vi "Plugin Main - Desaccade time data.vi"(7 "Background Mode":bool, 9 "threshold":dbl(slide) scale=0.0..500.0, 11 "Shared Data from EMA":T2={"Impulse Positions"=[], "Parameter Impuls Series"=[], "Data File"={"Data Channels"=[], "Sample Rate"=0, "Channel List"=[]}, "desacc "={"Threshold 1 [Acc]"=7000.0, "Threshold 2 [% of TH1]"=60, "tolerance"=3, "Search WD "=0.1, " always use TH2"=FALSE, "Range"=2.0, "Max time"=120.0, "Min time"=20.0, "Velocity Threshold"=150}, "Experiment Parameters 2"={"Subject"="", "Strain"="", "Rotation plane"="", "Experimenter"="", "Trial"=0.0, "Time"=0.0}} {"Parameter Impuls Series"."Gain" format="%.1f"; "Parameter Impuls Series"."Offset" format="%.1f"}) -> (3 "Shared Data from EMA 2":T2={"Impulse Positions"=[], "Parameter Impuls Series"=[], "Data File"={"Data Channels"=[], "Sample Rate"=0, "Channel List"=[]}, "desacc "={"Threshold 1 [Acc]"=7000.0, "Threshold 2 [% of TH1]"=60, "tolerance"=3, "Search WD "=0.1, " always use TH2"=FALSE, "Range"=2.0, "Max time"=120.0, "Min time"=20.0, "Velocity Threshold"=150}, "Experiment Parameters 2"={"Subject"="", "Strain"="", "Rotation plane"="", "Experimenter"="", "Trial"=0.0, "Time"=0.0}} {"Parameter Impuls Series"."Gain" format="%.1f"; "Parameter Impuls Series"."Offset" format="%.1f"})   [LabVIEW 2016]
uses:
  Plugin Shared Data.ctl
  core/type-defs/TD_Impulse Parameter.ctl
  <vilib>/Analysis/1siggen.llb/Ramp Pattern by Samples.vi
  <vilib>/Analysis/NI_AALBase.lvlib
  <vilib>/ptbypt/NI_PtbyPt.lvlib
  core/core.lvlib
  plugin data.lvlib
panel:
  out "XY Graph":T1(graph)
  in  "min delta Position for Quick-Phase":dbl=0.01
  in  "+/- # points post":i32
  in  "Time [ms]":dbl=60.0
  in  "Preview delete":bool
  in  "+/- # points pre":i32
  in  "Eye":enum16{"Right", "Left"}(ring)=enum."Left"
  in  "Pos/Vel":enum16{"Position", "Velocity"}(ring)=enum."Velocity"
  in  "Stop Button":bool
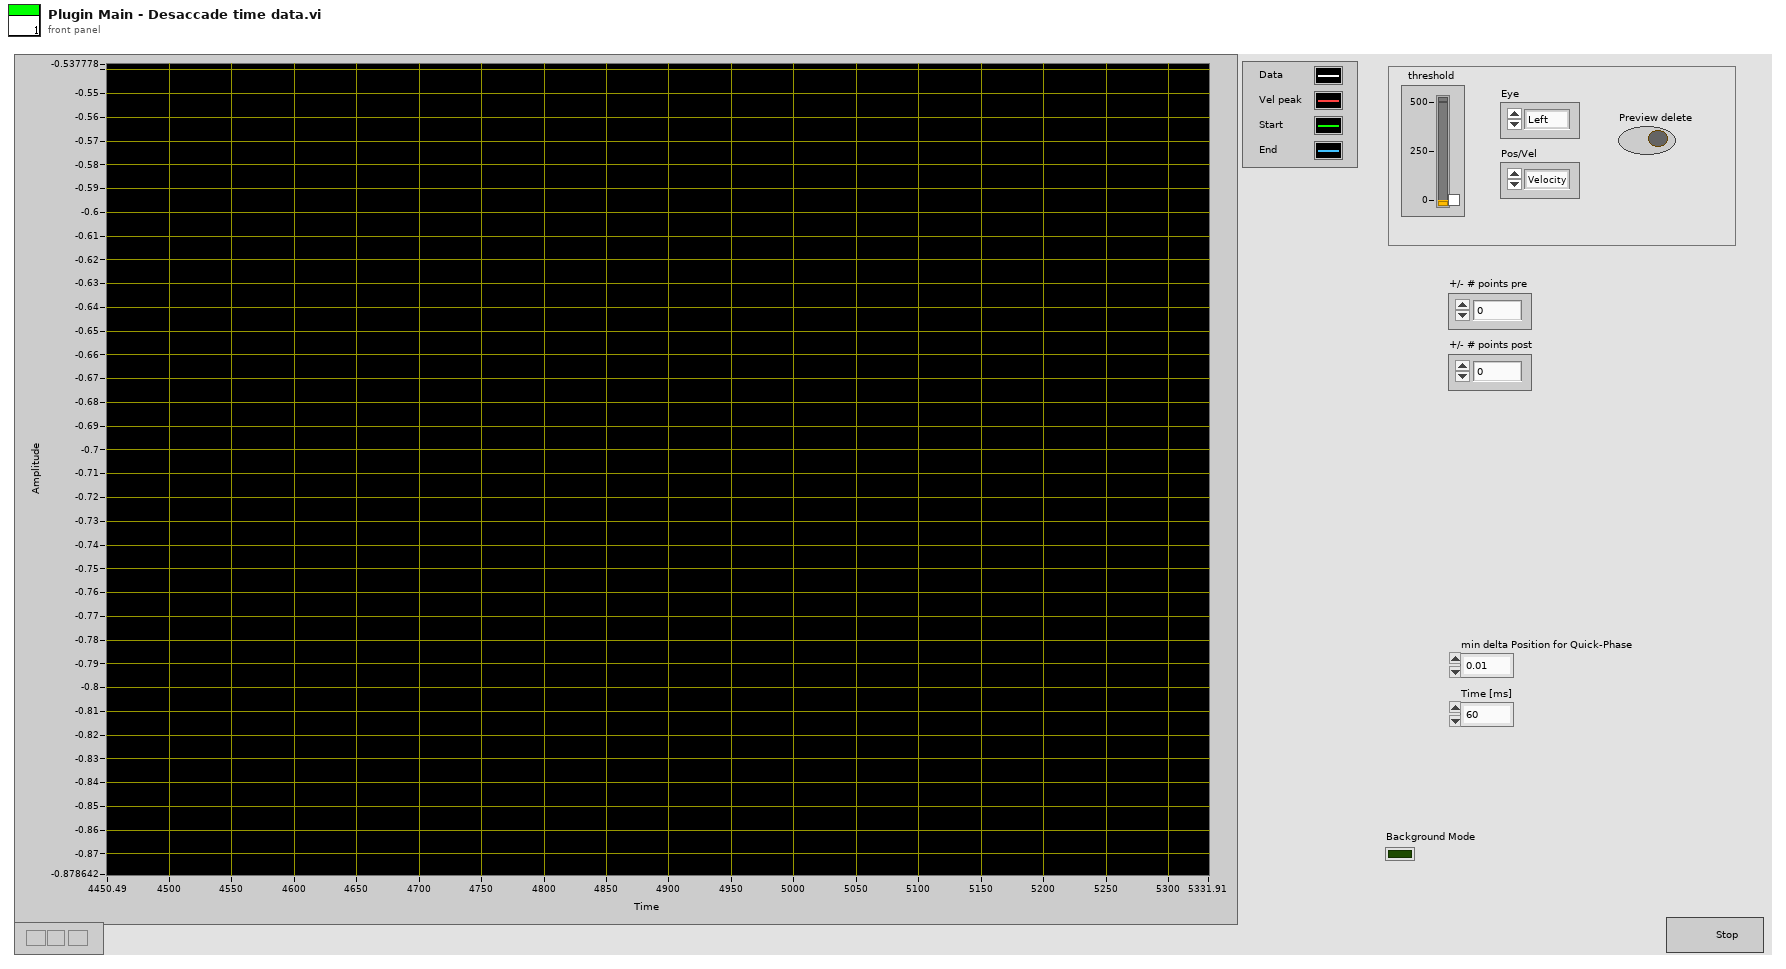
[diagram p1: front panel]
types:
  T1 = cluster{"Ramp Pattern":dbl[], "Data Channels":dbl[]}[]
  T2 = typedef "plugin data.lvlib/Plugin Shared Data.ctl" = cluster{"Impulse Positions":cluster{"Start":i32, "End":i32, "Impulse Plane":enum16{"Other", "Yaw", "Pitch", "Roll", "LARP", "RALP"}, "Impulse Direction +ve?":bool, "Time offset":i32, "Amplitude offset":dbl}[], "Parameter Impuls Series":T3, "Data File":cluster{"Data Channels":dbl[][], "Sample Rate":i32, "Channel List":string[]}, "desacc ":cluster{"Threshold 1 [Acc]":dbl, "Threshold 2 [% of TH1]":i32, "tolerance":i32, "Search WD ":dbl, " always use TH2":bool, "Range":dbl, "Max time":dbl, "Min time":dbl, "Velocity Threshold":i32}, "Experiment Parameters 2":cluster{"Subject":string, "Strain":string, "Rotation plane":string, "Experimenter":string, "Trial":dbl, "Time":dbl}}
  T3 = typedef "core.lvlib/TD_Impulse Parameter.ctl" = cluster{"Color":u32, "Visible":bool, "Channel":u16, "Invert":bool, "Desaccade":bool, "Offset":dbl, "Gain":dbl}[]
  T4 = cluster{"Channel Groups":i32[][][], "Saccade pos tmp":i32[], "Saccade dir":bool[], "newData":dbl[][], "Eye":enum16{"Right", "Left"}, "Saccade start tmp":i32[], "Saccade end tmp":i32[], "Saccades R":cluster{"Saccade pos":i32[], "Saccade start":i32[], "Saccade end":i32[]}, "Saccades L":cluster{"Saccade pos":i32[], "Saccade start":i32[], "Saccade end":i32[]}}
  T5 = cluster{"Ramp Pattern":dbl[], "Data Channels":dbl[]}
  T6 = cluster{"+/- # points pre":i32, "+/- # points post":i32, "threshold":dbl}
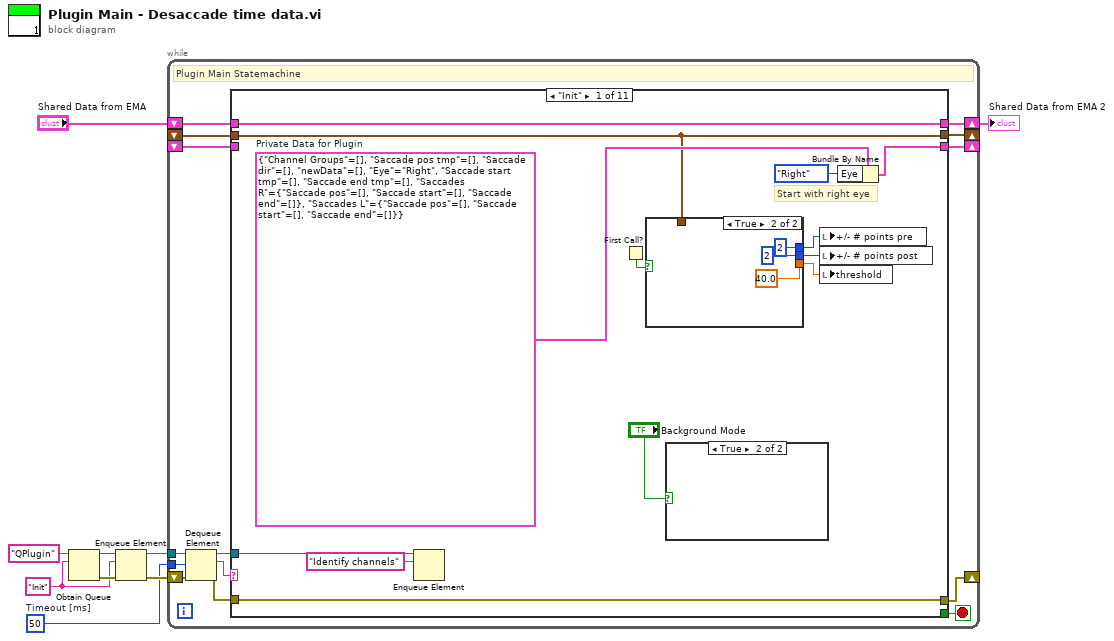
[diagram p0: block diagram]
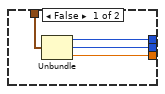
[diagram p2: hidden frame]
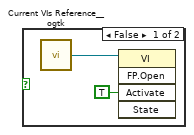
[diagram p3: hidden frame]
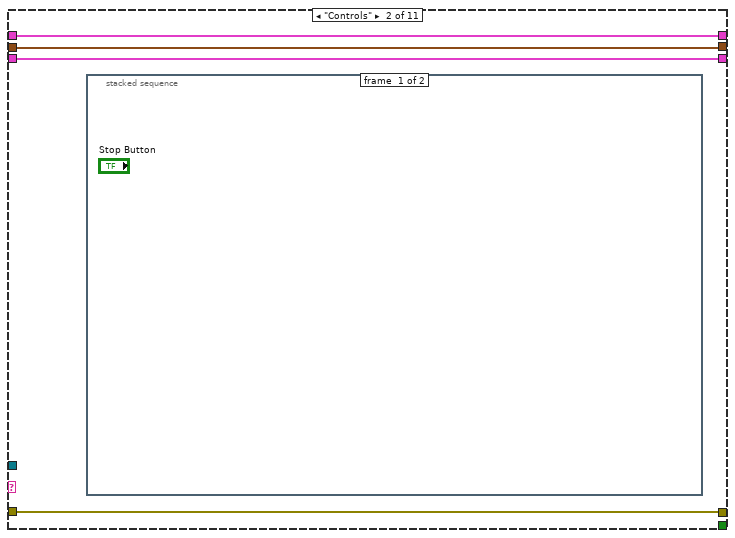
[diagram p4: hidden frame]
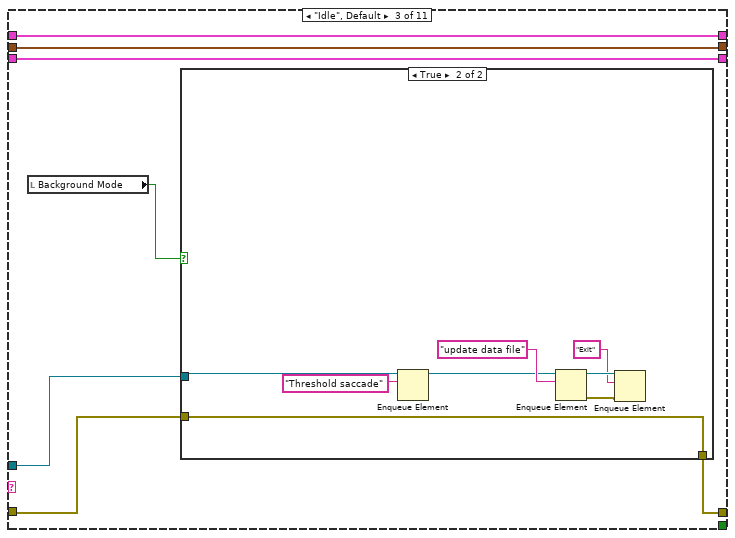
[diagram p6: hidden frame]
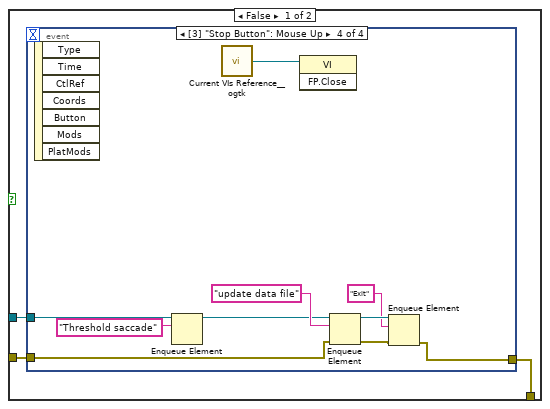
[diagram p7: hidden frame]
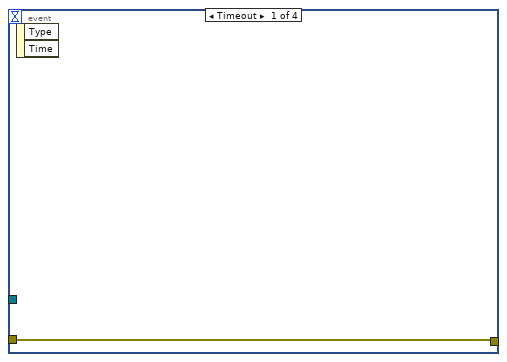
[diagram p8: hidden frame]
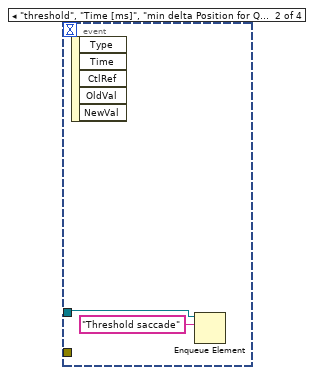
[diagram p9: hidden frame]
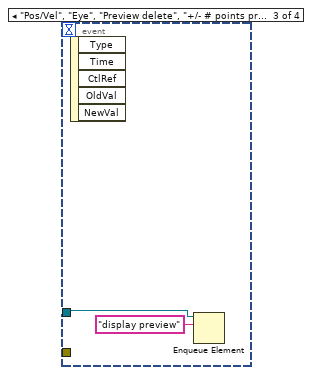
[diagram p10: hidden frame]
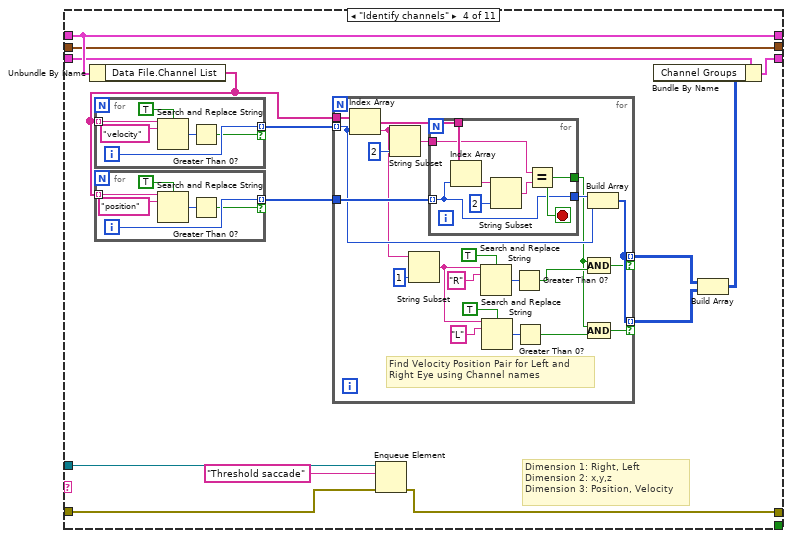
[diagram p11: hidden frame]
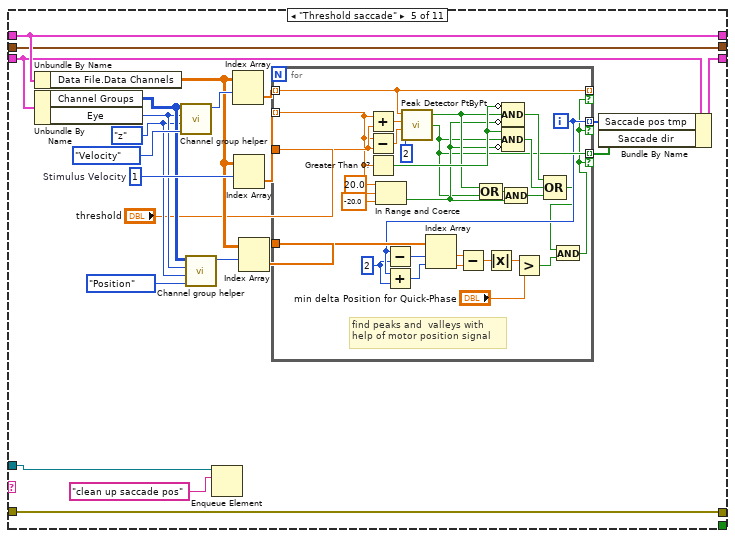
[diagram p12: hidden frame]
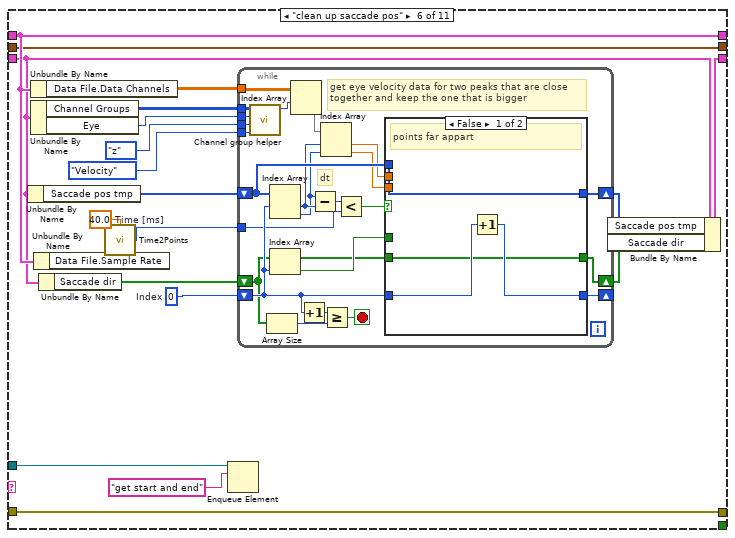
[diagram p13: hidden frame]
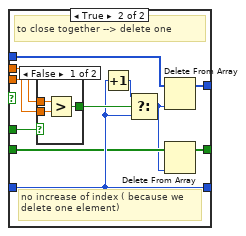
[diagram p14: hidden frame]
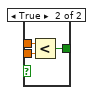
[diagram p15: hidden frame]
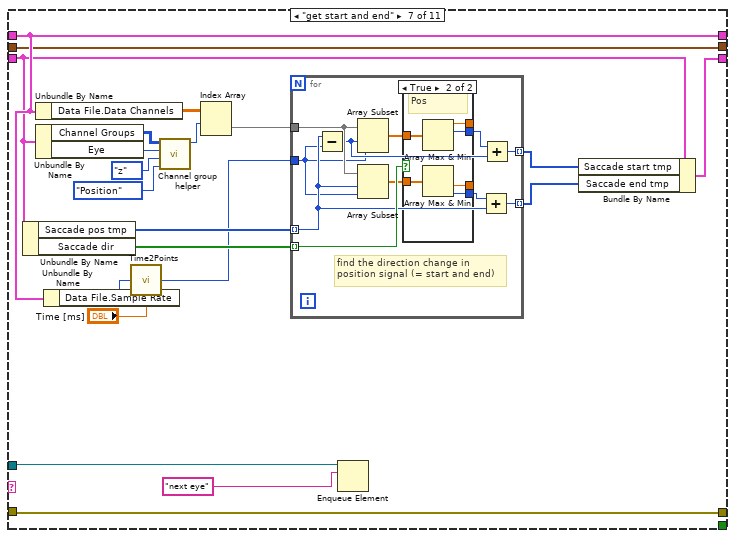
[diagram p16: hidden frame]
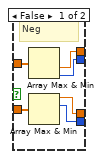
[diagram p17: hidden frame]
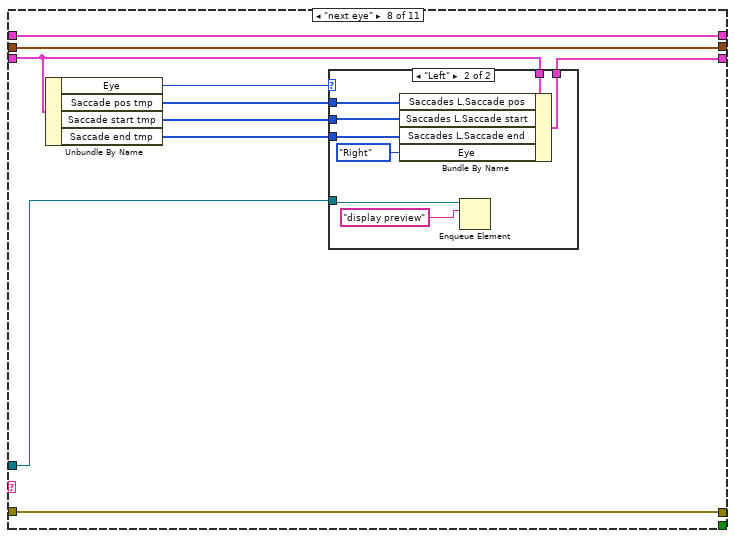
[diagram p18: hidden frame]
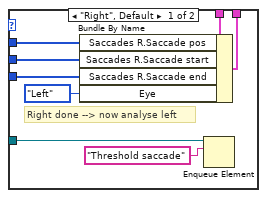
[diagram p19: hidden frame]
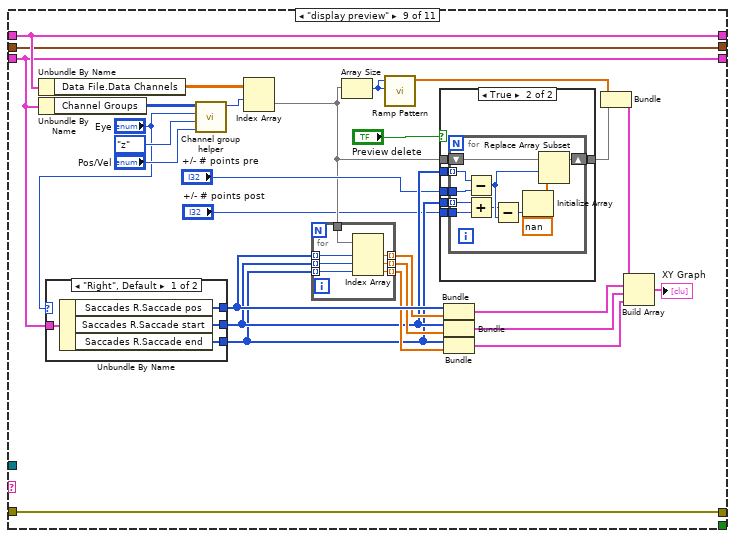
[diagram p20: hidden frame]
diagram:
  w3 = 50  # Timeout [ms]
  w7 = "Init"
  n1 = Obtain Queue(name (unnamed)="QPlugin", element data type=w7) -> (queue out=w8:refnum<queue>, error out=w9:errorcluster)  [unwired: 3 in, 1 out]
  n2 = Enqueue Element(queue=w8, element=w7, error in (no error)=w9) -> (queue out=w5:refnum<queue>, error out=w4:errorcluster)  [unwired: 1 in, 1 out]
  n3 = while {
    tunnel: w5 -> [w22]
    tunnel: w3 -> [w20]
    shift-right: [w16] -> _
    shift-left: w4 -> [w21]
    shift-right: [w15] -> _
    shift-left: _ -> [w14]
    shift-right: [w12] -> w1
    shift-left: "Shared Data from EMA" -> [w13]
    shift-right: [w11] -> _
    shift-left: _ -> [w10]
    stop <- w23 stop-if-true
    # "Plugin Main Statemachine"
    n4 = Dequeue Element(queue=w22, timeout in ms (-1)=w20, error in (no error)=w21) -> (queue out=w19:refnum<queue>, element=w18:string, error out=w17:errorcluster)  [unwired: 1 out]
    n5 = case shown="\"Init\"" w18 {
      tunnel: [_ _ _ _ _ _ _ _ _ _ w451] -> w23
      tunnel: w19 -> [w35 _ w54 w86 w154 w205 w256 w298 _ _ _]
      tunnel: w17 -> [w36 w47 w53 w85 w158 w207 w273 w305 w350 w391 w450]
      tunnel: [w36 w47 w52 w84 w158 w207 w273 w305 w350 w391 w450] -> w16
      tunnel: [w32 w48 w56 w88 w155 w199 w258 w299 w343 w388 w449] -> w15
      tunnel: w14 -> [_ w48 w56 w89 w156 w191 w259 w300 w343 w388 w449]
      tunnel: w13 -> [w30 w49 w55 w96 w157 w195 w263 w306 w349 w387 w448]
      tunnel: [w30 w49 w55 w96 w157 w195 w263 w306 w349 w386 w448] -> w12
      tunnel: [w25 w46 w50 w83 w137 w188 w253 w297 w323 w384 w444] -> w11
      tunnel: w10 -> [w25 w46 w50 w83 w137 w188 w253 w297 w323 w384 _]
      frame "Init" {
        w33 = T4 {"Channel Groups"=[], "Saccade pos tmp"=[], "Saccade dir"=[], "newData"=[], "Eye"=enum."Right", "Saccade start tmp"=[], "Saccade end tmp"=[], "Saccades R"={"Saccade pos"=[], "Saccade start"=[], "Saccade end"=[]}, "Saccades L"={"Saccade pos"=[], "Saccade start"=[], "Saccade end"=[]}}  # Private Data for Plugin
        # "Start with right eye"
        n6 = Enqueue Element(queue=w35, element="Identify channels") -> ()  [unwired: 2 in, 3 out]
        n7 = First Call?() -> (First Call?: T/F=w24:bool)
        n8 = case shown="True" w24 {
          tunnel: [w40 2 ("+/- # points pre")] -> w28
          tunnel: [w39 2 ("+/- # points post")] -> w27
          tunnel: [w38 40.0 ("threshold")] -> w26
          tunnel: w25 -> [w37 _]
          frame False {
            n9 = Unbundle(w37) -> ("+/- # points pre"=w40:i32, "+/- # points post"=w39:i32, "threshold"=w38:dbl)
          }
          frame True {
          }
        }
        n10 = case shown="True" "Background Mode" {
          frame False {
            n11 = call <userlib>:"Current VIs Reference__ogtk.vi"() -> ("Current VI's reference"=w45:refnum<vi>)  [unwired: 5 in]
            n12 = invoke class="VI" method="FP.Open"(reference=w45, "Activate"=TRUE ("Activate?")) -> ()  [unwired: 3 in, 5 out]
          }
          frame True {
          }
        }
        n13 = local write "+/- # points pre"(w28) -> ()
        n14 = local write "+/- # points post"(w27) -> ()
        n15 = local write "threshold"(w26) -> ()
        n16 = Bundle By Name(cluster=w33, "Eye"=enum16{"Right", "Left"}."Right") -> (w32:T4)
      }
      frame "Controls" {
        n17 = stacked-sequence {
          frame #0 {
          }
          frame #1 {
          }
        }
      }
      frame "Idle", Default {
        n18 = local read "Background Mode"() -> (w51:bool)
        n19 = case shown="True" w51 {
          tunnel: w54 -> [w59 w75]
          tunnel: w53 -> [w58 w82]
          tunnel: [w57 w82] -> w52
          frame False {
            n20 = event shown="[3] \"Stop Button\": Mouse Up" {
              selector: _ -> [_ _ _ _]
              dyn-events: _ -> [_ _ _ _]
              timeout: _ -> [_ _ _ _]
              tunnel: w59 -> [_ w61 w63 w67]
              tunnel: w58 -> [w60 _ _ w73]
              tunnel: [w60 _ _ w70] -> w57
              event Timeout {
                n21 = event-data() -> ()  [unwired: 1 in, 2 out]
              }
              event "threshold", "Time [ms]", "min delta Position for Quick-Phase": Value Change {
                n22 = event-data() -> ()  [unwired: 1 in, 5 out]
                n23 = Enqueue Element(queue=w61, element="Threshold saccade") -> ()  [unwired: 2 in, 3 out]
              }
              event "Pos/Vel", "Eye", "Preview delete", "+/- # points pre", "+/- # points post": Value Change {
                n24 = event-data() -> ()  [unwired: 1 in, 5 out]
                n25 = Enqueue Element(queue=w63, element="display preview") -> ()  [unwired: 2 in, 3 out]
              }
              event "Stop Button": Mouse Up {
                n26 = event-data() -> ()  [unwired: 1 in, 7 out]
                n27 = Enqueue Element(queue=w67, element="Threshold saccade") -> (queue out=w66:refnum<queue>)  [unwired: 2 in, 2 out]
                n28 = call <userlib>:"Current VIs Reference__ogtk.vi"() -> ("Current VI's reference"=w65:refnum<vi>)  [unwired: 5 in]
                n29 = invoke class="VI" method="FP.Close"(reference=w65) -> ()  [unwired: 2 in, 3 out]
                n30 = Enqueue Element(queue=w66, element="update data file", error in (no error)=w73) -> (queue out=w72:refnum<queue>, error out=w71:errorcluster)  [unwired: 1 in, 1 out]
                n31 = Enqueue Element(queue=w72, element="Exit", error in (no error)=w71) -> (error out=w70:errorcluster)  [unwired: 1 in, 2 out]
              }
            }
          }
          frame True {
            n32 = Enqueue Element(queue=w75, element="Threshold saccade") -> (queue out=w76:refnum<queue>)  [unwired: 2 in, 2 out]
            n33 = Enqueue Element(queue=w76, element="update data file") -> (queue out=w80:refnum<queue>, error out=w79:errorcluster)  [unwired: 2 in, 1 out]
            n34 = Enqueue Element(queue=w80, element="Exit", error in (no error)=w79) -> ()  [unwired: 1 in, 3 out]
          }
        }
      }
      frame "Identify channels" {
        # "Dimension 1: Right, Left\nDimension 2: x,y,z\nDimension 3: Position, Velocity"
        n35 = Unbundle By Name(w96) -> ("Data File.Channel List"=w93:string[])
        n36 = for {
          tunnel: w93 -> [w136] mode=indexing
          tunnel: [w133] -> w95 mode=indexing if=w132
          i -> [w133]
          n37 = Search and Replace String(case sensitive?=TRUE ("ignore case? (F)"), input string=w136, search string="velocity") -> (number of replacements=w134:i32)  [unwired: 5 in, 3 out]
          n38 = Greater Than 0?(x=w134) -> (x > 0?=w132:bool)
        }
        n39 = for {
          tunnel: w93 -> [w130] mode=indexing
          tunnel: [w127] -> w94 mode=indexing if=w126
          i -> [w127]
          n40 = Search and Replace String(case sensitive?=TRUE ("ignore case? (F)"), input string=w130, search string="position") -> (number of replacements=w128:i32)  [unwired: 5 in, 3 out]
          n41 = Greater Than 0?(x=w128) -> (x > 0?=w126:bool)
        }
        n42 = for {
          tunnel: w95 -> [w112] mode=indexing
          tunnel: w93 -> [w116]
          tunnel: w94 -> [w117]
          tunnel: [w108] -> w92 mode=indexing if=w98
          tunnel: [w108] -> w91 mode=indexing if=w97
          # "Find Velocity Position Pair for Left and \nRight Eye using Channel names"
          n43 = Index Array(array=w116, index=w112) -> (element=w100:string)
          n44 = String Subset(string=w100, length (rest)=2 ("length (rest)")) -> (substring=w114:string)  [unwired: 1 in]
          n45 = String Subset(string=w100, length (rest)=1 ("length (rest)")) -> (substring=w104:string)  [unwired: 1 in]
          n46 = for {
            tunnel: w117 -> [w118] mode=indexing
            tunnel: w116 -> [w123]
            tunnel: w114 -> [w120]
            tunnel: [w119] -> w102
            tunnel: [w118] -> w113
            stop <- w119 stop-if-true
            n47 = Index Array(array=w123, index=w118) -> (element=w124:string)
            n48 = String Subset(string=w124, length (rest)=2 ("length (rest)")) -> (substring=w121:string)  [unwired: 1 in]
            n49 = Equal?(x=w120, y=w121) -> (x = y?=w119:bool)
          }
          n50 = Search and Replace String(case sensitive?=TRUE ("ignore case? (F)"), input string=w104, search string="R") -> (number of replacements=w109:i32)  [unwired: 5 in, 3 out]
          n51 = Search and Replace String(case sensitive?=TRUE ("ignore case? (F)"), input string=w104, search string="L") -> (number of replacements=w107:i32)  [unwired: 5 in, 3 out]
          n52 = Greater Than 0?(x=w109) -> (x > 0?=w103:bool)
          n53 = Greater Than 0?(x=w107) -> (x > 0?=w101:bool)
          n54 = Build Array(w113, w112) -> (w108:i32[])
          n55 = Compound Arithmetic op=AND(w102, w103) -> (w98:bool)
          n56 = Compound Arithmetic op=AND(w102, w101) -> (w97:bool)
        }
        n57 = Enqueue Element(queue=w86, element="Threshold saccade", error in (no error)=w85) -> (error out=w84:errorcluster)  [unwired: 1 in, 2 out]
        n58 = Build Array(w92, w91) -> (w90:i32[][][])
        n59 = Bundle By Name(cluster=w89, "Channel Groups"=w90) -> (w88:T4)
      }
      frame "Threshold saccade" {
        w140 = enum16{"x", "y", "z"}."z" ("Eye component")
        w151 = 1  # Stimulus Velocity
        n60 = Unbundle By Name(w157) -> ("Data File.Data Channels"=w145:dbl[][])
        n61 = Unbundle By Name(w156) -> ("Channel Groups"=w142:i32[][][], "Eye"=w141:enum16{"Right", "Left"})
        n62 = call "Channel group helper.vi"("Pos/Vel"=enum16{"Position", "Velocity"}."Velocity", "Eye component"=w140, "Eye"=w141, "Channel Groups"=w142) -> ("Channel"=w149:i32)  [unwired: 7 in]
        n63 = call "Channel group helper.vi"("Pos/Vel"=enum16{"Position", "Velocity"}."Position", "Eye component"=w140, "Eye"=w141, "Channel Groups"=w142) -> ("Channel"=w144:i32)  [unwired: 7 in]
        n64 = Enqueue Element(queue=w154, element="clean up saccade pos") -> ()  [unwired: 2 in, 3 out]
        n65 = Index Array(array=w145, index (row)=w149) -> (element=w147:dbl[])  [unwired: 1 in]
        n66 = Index Array(array=w145, index (row)=w151) -> (element=w146:dbl[])  [unwired: 1 in]
        n67 = Index Array(array=w145, index (row)=w144) -> (element=w143:dbl[])  [unwired: 1 in]
        n68 = for {
          tunnel: w147 -> [w187] mode=indexing
          tunnel: w146 -> [w180] mode=indexing
          tunnel: "threshold" -> [w184]
          tunnel: [w187] -> _ mode=indexing if=w159
          tunnel: [w170] -> w150 mode=indexing if=w159
          tunnel: [w172] -> w152 mode=indexing if=w159
          tunnel: w143 -> [w171]
          i -> [w170]
          w169 = 2 ("y")
          # "find peaks and  valleys with \nhelp of motor position signal"
          n69 = Add(x=w180, y=w184) -> (x+y=w183:dbl)
          n70 = Subtract(x=w180, y=w184) -> (x-y=w182:dbl)
          n71 = Greater Than 0?(x=w180) -> (x > 0?=w177:bool)
          n72 = In Range and Coerce(upper limit=20.0, x=w180, lower limit=-20.0) -> (In Range?=w174:bool)  [unwired: 1 out]
          n73 = Subtract(x=w170, y=w169) -> (x-y=w168:i32)
          n74 = Add(x=w170, y=w169) -> (x+y=w167:i32)
          n75 = call <vilib>:"Peak Detector PtByPt.vi"("x"=w187, "threshold peak"=w183, "threshold valley"=w182, "width"=2) -> ("peak"=w176:bool, "valley"=w172:bool)  [unwired: 1 in, 1 out]
          n76 = Index Array(array=w171, index #1=w168, index #2=w167) -> (element #1=w166:dbl, element #2=w165:dbl)
          n77 = Subtract(x=w166, y=w165) -> (x-y=w164:dbl)
          n78 = Compound Arithmetic op=OR(w176, w172) -> (w175:bool)
          n79 = Absolute Value(x=w164) -> (abs(x)=w163:dbl)
          n80 = Compound Arithmetic op=AND(invert w177, w176, invert w174) -> (w185:bool)
          n81 = Compound Arithmetic op=AND(w177, w172, invert w174) -> (w181:bool)
          n82 = Compound Arithmetic op=AND(w175, w174) -> (w173:bool)
          n83 = Greater?(x=w163, y="min delta Position for Quick-Phase") -> (0:w160:bool)
          n84 = Compound Arithmetic op=OR(w185, w181, w173) -> (w161:bool)
          n85 = And(x=w161, y=w160) -> (x .and. y?=w159:bool)
        }
        n86 = Bundle By Name(cluster=w156, "Saccade pos tmp"=w150, "Saccade dir"=w152) -> (w155:T4)
      }
      frame "clean up saccade pos" {
        w193 = 40.0  # Time [ms]
        w203 = 0  # Index
        n87 = Unbundle By Name(w191) -> ("Saccade pos tmp"=w204:i32[])
        n88 = Unbundle By Name(w195) -> ("Data File.Data Channels"=w202:dbl[][])
        n89 = Unbundle By Name(w191) -> ("Channel Groups"=w198:i32[][][], "Eye"=w197:enum16{"Right", "Left"})
        n90 = Unbundle By Name(w195) -> ("Data File.Sample Rate"=w194:i32)
        n91 = Unbundle By Name(w191) -> ("Saccade dir"=w190:bool[])
        n92 = call "Time2Points.vi"("Time [ms]"=w193, "Sample Rate"=w194) -> ("Points"=w192:i32)  [unwired: 2 in]
        n93 = Enqueue Element(queue=w205, element="get start and end") -> ()  [unwired: 2 in, 3 out]
        n94 = while {
          shift-right: [w225] -> w201
          shift-left: w204 -> [w228]
          shift-right: [w229] -> _
          shift-left: w203 -> [w221]
          tunnel: w202 -> [w214]
          shift-right: [w223] -> w200
          shift-left: w190 -> [w219]
          tunnel: w198 -> [w213]
          tunnel: w197 -> [w210]
          tunnel: enum16{"Position", "Velocity"}."Velocity" ("Pos/Vel") -> [w212]
          tunnel: w192 -> [w220]
          tunnel: enum16{"x", "y", "z"}."z" ("Eye component") -> [w211]
          stop <- w226 stop-if-true
          # "dt"
          # "get eye velocity data for two peaks that are close\ntogether and keep the one that is bigger"
          n95 = call "Channel group helper.vi"("Pos/Vel"=w212, "Eye component"=w211, "Eye"=w210, "Channel Groups"=w213) -> ("Channel"=w209:i32)  [unwired: 7 in]
          n96 = Array Size(array=w219) -> (size(s)=w227:i32)
          n97 = Index Array(array=w228, index #1=w221) -> (element #1=w218:i32, element #2=w217:i32)  [unwired: 1 in]
          n98 = Index Array(array=w219, index=w221) -> (element=w222:bool)
          n99 = Index Array(array=w214, index (row)=w209) -> (element=w208:dbl[])  [unwired: 1 in]
          n100 = Increment(x=w221) -> (x+1=w224:i32)
          n101 = Subtract(x=w217, y=w218) -> (x-y=w231:i32)
          n102 = Index Array(array=w208, index #1=w218, index #2=w217) -> (element #1=w216:dbl, element #2=w215:dbl)
          n103 = Greater Or Equal?(x=w224, y=w227) -> (x >= y?=w226:bool)
          n104 = Less?(x=w231, y=w220) -> (x < y?=w230:bool)
          n105 = case shown="False" w230 {
            tunnel: w216 -> [_ w246]
            tunnel: w215 -> [_ w245]
            tunnel: w221 -> [w234 w240]
            tunnel: [w235 w243] -> w225
            tunnel: w228 -> [w235 w242]
            tunnel: [w233 w240] -> w229
            tunnel: w219 -> [w232 w239]
            tunnel: [w232 w238] -> w223
            tunnel: w222 -> [_ w237]
            frame False {
              # "points far appart"
              n106 = Increment(x=w234) -> (x+1=w233:i32)
            }
            frame True {
              # "no increase of index ( because we \ndelete one element)"
              # "to close together --> delete one"
              n107 = case shown="False" w237 {
                tunnel: w246 -> [w249 w252]
                tunnel: w245 -> [w248 w251]
                tunnel: [w247 w250] -> w244
                frame False {
                  n108 = Greater?(x=w249, y=w248) -> (0:w247:bool)
                }
                frame True {
                  n109 = Less?(x=w252, y=w251) -> (x < y?=w250:bool)
                }
              }
              n110 = Increment(x=w240) -> (x+1=w241:i32)
              n111 = Select(t=w241, s=w244, f=w240) -> (s? t:f=w236:i32)
              n112 = Delete From Array(array=w242, index=w236) -> (array with subset deleted=w243:i32[])  [unwired: 1 in, 1 out]
              n113 = Delete From Array(array=w239, index=w236) -> (array with subset deleted=w238:bool[])  [unwired: 1 in, 1 out]
            }
          }
        }
        n114 = Bundle By Name(cluster=w191, "Saccade pos tmp"=w201, "Saccade dir"=w200) -> (w199:T4)
      }
      frame "get start and end" {
        n115 = Unbundle By Name(w259) -> ("Saccade pos tmp"=w272:i32[], "Saccade dir"=w271:bool[])
        n116 = Unbundle By Name(w263) -> ("Data File.Data Channels"=w269:dbl[][])
        n117 = Unbundle By Name(w259) -> ("Channel Groups"=w268:i32[][][], "Eye"=w267:enum16{"Right", "Left"})
        n118 = Unbundle By Name(w263) -> ("Data File.Sample Rate"=w262:i32)
        n119 = call "Time2Points.vi"("Time [ms]"="Time [ms]", "Sample Rate"=w262) -> ("Points"=w260:i32)  [unwired: 2 in]
        n120 = call "Channel group helper.vi"("Pos/Vel"=enum16{"Position", "Velocity"}."Position", "Eye component"=enum16{"x", "y", "z"}."z", "Eye"=w267, "Channel Groups"=w268) -> ("Channel"=w265:i32)  [unwired: 7 in]
        n121 = Index Array(array=w269, index (row)=w265) -> (element=w270:dbl[])  [unwired: 1 in]
        n122 = for {
          tunnel: w272 -> [w275] mode=indexing
          tunnel: w270 -> [w279]
          tunnel: [w282] -> w255 mode=indexing
          tunnel: [w281] -> w254 mode=indexing
          tunnel: w271 -> [w278] mode=indexing
          tunnel: w260 -> [w274]
          # "find the direction change in \nposition signal (= start and end)"
          n123 = Subtract(x=w275, y=w274) -> (x-y=w276:i32)
          n124 = Array Subset(array=w279, index=w276, length=w274) -> (w284:dbl[])
          n125 = Array Subset(array=w279, index=w275, length=w274) -> (w277:dbl[])
          n126 = case shown="True" w278 {
            tunnel: w284 -> [w290 w296]
            tunnel: [w288 w291] -> w283
            tunnel: [w289 w292] -> _
            tunnel: [w286 w294] -> _
            tunnel: [w285 w293] -> w280
            tunnel: w277 -> [w287 w295]
            frame False {
              # "Neg"
              n127 = Array Max & Min(array=w290) -> (min value=w289:dbl, min index (indices)=w288:i32)  [unwired: 2 out]
              n128 = Array Max & Min(array=w287) -> (max value=w286:dbl, max index (indices)=w285:i32)  [unwired: 2 out]
            }
            frame True {
              # "Pos"
              n129 = Array Max & Min(array=w296) -> (max value=w292:dbl, max index (indices)=w291:i32)  [unwired: 2 out]
              n130 = Array Max & Min(array=w295) -> (min value=w294:dbl, min index (indices)=w293:i32)  [unwired: 2 out]
            }
          }
          n131 = Add(x=w280, y=w275) -> (x+y=w281:i32)
          n132 = Add(x=w283, y=w276) -> (x+y=w282:i32)
        }
        n133 = Enqueue Element(queue=w256, element="next eye") -> ()  [unwired: 2 in, 3 out]
        n134 = Bundle By Name(cluster=w259, "Saccade start tmp"=w255, "Saccade end tmp"=w254) -> (w258:T4)
      }
      frame "next eye" {
        n135 = Unbundle By Name(w300) -> ("Eye"=w304:enum16{"Right", "Left"}, "Saccade pos tmp"=w303:i32[], "Saccade start tmp"=w302:i32[], "Saccade end tmp"=w301:i32[])
        n136 = case shown="\"Left\"" w304 {
          tunnel: w300 -> [w314 w322]
          tunnel: w303 -> [w313 w320]
          tunnel: w302 -> [w312 w319]
          tunnel: w301 -> [w311 w318]
          tunnel: [w310 w321] -> w299
          tunnel: w298 -> [w308 w316]
          frame "Right", Default {
            # "Right done --> now analyse left"
            n137 = Bundle By Name(cluster=w314, "Saccades R.Saccade pos"=w313, "Saccades R.Saccade start"=w312, "Saccades R.Saccade end"=w311, "Eye"=enum16{"Right", "Left"}."Left") -> (w310:T4)
            n138 = Enqueue Element(queue=w308, element="Threshold saccade") -> ()  [unwired: 2 in, 3 out]
          }
          frame "Left" {
            n139 = Bundle By Name(cluster=w322, "Saccades L.Saccade pos"=w320, "Saccades L.Saccade start"=w319, "Saccades L.Saccade end"=w318, "Eye"=enum16{"Right", "Left"}."Right") -> (w321:T4)
            n140 = Enqueue Element(queue=w316, element="display preview") -> ()  [unwired: 2 in, 3 out]
          }
        }
      }
      frame "display preview" {
        n141 = Unbundle By Name(w349) -> ("Data File.Data Channels"=w348:dbl[][])
        n142 = Unbundle By Name(w343) -> ("Channel Groups"=w347:i32[][][])
        n143 = case shown="\"Right\", Default" "Eye" {
          tunnel: w343 -> [w372 w376]
          tunnel: [w371 w375] -> w342
          tunnel: [w370 w374] -> w330
          tunnel: [w369 w373] -> w329
          frame "Right", Default {
            n144 = Unbundle By Name(w372) -> ("Saccades R.Saccade pos"=w371:i32[], "Saccades R.Saccade start"=w370:i32[], "Saccades R.Saccade end"=w369:i32[])
          }
          frame "Left" {
            n145 = Unbundle By Name(w376) -> ("Saccades L.Saccade pos"=w375:i32[], "Saccades L.Saccade start"=w374:i32[], "Saccades L.Saccade end"=w373:i32[])
          }
        }
        n146 = call "Channel group helper.vi"("Pos/Vel"="Pos/Vel", "Eye component"=enum16{"x", "y", "z"}."z", "Eye"="Eye", "Channel Groups"=w347) -> ("Channel"=w346:i32)  [unwired: 7 in]
        n147 = Index Array(array=w348, index (row)=w346) -> (element=w327:dbl[])  [unwired: 1 in]
        n148 = for {
          tunnel: w327 -> [w383]
          tunnel: w342 -> [w382] mode=indexing
          tunnel: w330 -> [w381] mode=indexing
          tunnel: w329 -> [w380] mode=indexing
          tunnel: [w379] -> w341 mode=indexing
          tunnel: [w378] -> w340 mode=indexing
          tunnel: [w377] -> w339 mode=indexing
          n149 = Index Array(array=w383, index #1=w382, index #2=w381, index #3=w380) -> (element #1=w379:dbl, element #2=w378:dbl, element #3=w377:dbl)
        }
        n150 = Array Size(array=w327) -> (size(s)=w332:i32)
        n151 = call-poly <vilib>:"Ramp Pattern.vi"("end"=w332, "samples"=w332) -> ("Ramp Pattern"=w338:dbl[])  [unwired: 8 in, 1 out]
        n152 = case shown="True" "Preview delete" {
          tunnel: w330 -> [_ w357]
          tunnel: w329 -> [_ w356]
          tunnel: "+/- # points pre" -> [_ w355]
          tunnel: w327 -> [w351 w354]
          tunnel: [w351 w353] -> w326
          tunnel: "+/- # points post" -> [_ w352]
          frame False {
          }
          frame True {
            n153 = for {
              shift-right: [w364] -> w353
              shift-left: w354 -> [w368]
              tunnel: w357 -> [w363] mode=indexing
              tunnel: w356 -> [w361] mode=indexing
              tunnel: w355 -> [w359]
              tunnel: w352 -> [w358]
              n154 = Subtract(x=w363, y=w359) -> (x-y=w362:i32)
              n155 = Add(x=w361, y=w358) -> (x+y=w360:i32)
              n156 = Subtract(x=w360, y=w362) -> (x-y=w367:i32)
              n157 = Initialize Array(nan ("element"), w367) -> (w365:dbl[])
              n158 = Replace Array Subset(array=w368, new element=w365, index=w362) -> (w364:dbl[])
            }
          }
        }
        n159 = Bundle("Saccade pos"=w342, w341) -> (w336:cluster{"Saccade pos":i32[], dbl[]})  [unwired: 1 in]
        n160 = Bundle("Saccade start"=w330, w340) -> (w335:cluster{"Saccade start":i32[], dbl[]})  [unwired: 1 in]
        n161 = Bundle("Saccade end"=w329, w339) -> (w334:cluster{"Saccade end":i32[], dbl[]})  [unwired: 1 in]
        n162 = Bundle("Ramp Pattern"=w338, "Data Channels"=w326) -> (w337:T5)  [unwired: 1 in]
        n163 = Build Array(w337, w336, w335, w334) -> (→"XY Graph":T1)
      }
      frame "update data file" {
        w389 = enum16{"Right", "Left"}[] [enum."Right", enum."Left"] items=["Right", "Left"]
        n164 = Unbundle By Name(w387) -> ("Data File.Data Channels"=w390:dbl[][])
        n165 = for {
          tunnel: w388 -> [w399]
          shift-right: [w393] -> w385
          shift-left: w390 -> [w400]
          tunnel: w389 -> [w396] mode=indexing
          tunnel: w388 -> [w395]
          w397 = enum16{"Position", "Velocity"}[] [enum."Position", enum."Velocity"] items=["Position", "Velocity"]
          w398 = enum16{"x", "y", "z"}[] [enum."x", enum."y", enum."z"] items=["x", "y", "z"]
          n166 = Unbundle By Name(w399) -> ("Channel Groups"=w403:i32[][][])
          n167 = case shown="\"Left\"" w396 {
            tunnel: [w440 w443] -> w402
            tunnel: [w439 w442] -> w401
            tunnel: w395 -> [w438 w441]
            frame "Right", Default {
              n168 = Unbundle By Name(w438) -> ("Saccades R.Saccade start"=w440:i32[], "Saccades R.Saccade end"=w439:i32[])
            }
            frame "Left" {
              n169 = Unbundle By Name(w441) -> ("Saccades L.Saccade start"=w443:i32[], "Saccades L.Saccade end"=w442:i32[])
            }
          }
          n170 = local read "+/- # points pre"() -> (w394:i32)
          n171 = local read "+/- # points post"() -> (w392:i32)
          n172 = for {
            tunnel: w403 -> [w413]
            tunnel: w402 -> [w412]
            tunnel: w401 -> [w411]
            shift-right: [w409] -> w393
            shift-left: w400 -> [w410]
            tunnel: w398 -> [w408]
            tunnel: w397 -> [w407] mode=indexing
            tunnel: w396 -> [w406]
            tunnel: w394 -> [w405]
            tunnel: w392 -> [w404]
            n173 = for {
              tunnel: w413 -> [w426]
              tunnel: w412 -> [w425]
              tunnel: w411 -> [w424]
              shift-right: [w419] -> w409
              shift-left: w410 -> [w422]
              tunnel: w408 -> [w418] mode=indexing
              tunnel: w407 -> [w417]
              tunnel: w406 -> [w416]
              tunnel: w405 -> [w415]
              tunnel: w404 -> [w414]
              n174 = call "Channel group helper.vi"("Pos/Vel"=w417, "Eye component"=w418, "Eye"=w416, "Channel Groups"=w426) -> ("Channel"=w421:i32)  [unwired: 7 in]
              n175 = Index Array(array=w422, index (row)=w421) -> (element=w423:dbl[])  [unwired: 1 in]
              n176 = for {
                shift-right: [w433] -> w420
                shift-left: w423 -> [w437]
                tunnel: w425 -> [w430] mode=indexing
                tunnel: w424 -> [w429] mode=indexing
                tunnel: w415 -> [w428]
                tunnel: w414 -> [w427]
                n177 = Subtract(x=w430, y=w428) -> (x-y=w432:i32)
                n178 = Add(x=w429, y=w427) -> (x+y=w431:i32)
                n179 = Subtract(x=w431, y=w432) -> (x-y=w436:i32)
                n180 = Initialize Array(nan ("element"), w436) -> (w434:dbl[])
                n181 = Replace Array Subset(array=w437, new element=w434, index=w432) -> (w433:dbl[])
              }
              n182 = Replace Array Subset(array=w422, new element=w420, index (row)=w421) -> (w419:dbl[][])  [unwired: 1 in]
            }
          }
        }
        n183 = Bundle By Name(cluster=w387, "Data File.Data Channels"=w385) -> (w386:T2)
      }
      frame "Exit" {
        w451 = TRUE  # Quit Plugin
        n184 = local read "+/- # points pre"() -> (w445:i32)
        n185 = local read "+/- # points post"() -> (w446:i32)
        n186 = local read "threshold"() -> (w447:dbl)
        n187 = Bundle("+/- # points pre"=w445, "+/- # points post"=w446, "threshold"=w447) -> (w444:T6)  [unwired: 1 in]
      }
    }
  }
  "Shared Data from EMA 2" <- w1
